vi "test_voltage.vi"() -> ()   [LabVIEW 2017]
panel:
  out "Det P (uW)":string
  out "Inc P (uW)":string
  out "Inc V (CORRECTED)":dbl
  out "Det V (CORRECTED)":dbl
  out "Det V / Inc V (CORRECTED)":dbl
  out "Incident Voltage (mV)":dbl
  out "Detected Voltage (mV)":dbl
  in  "Detected Offset":dbl
  in  "Incident Offset":dbl
  out "Det P / Inc P":dbl
  in  "number of samples":i32=100
  in  "rate":dbl=100.0
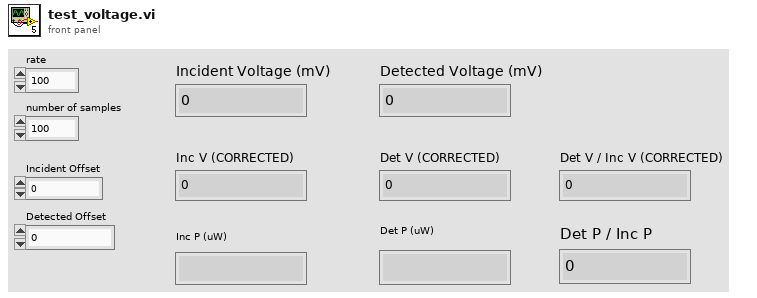
[diagram p1: front panel]
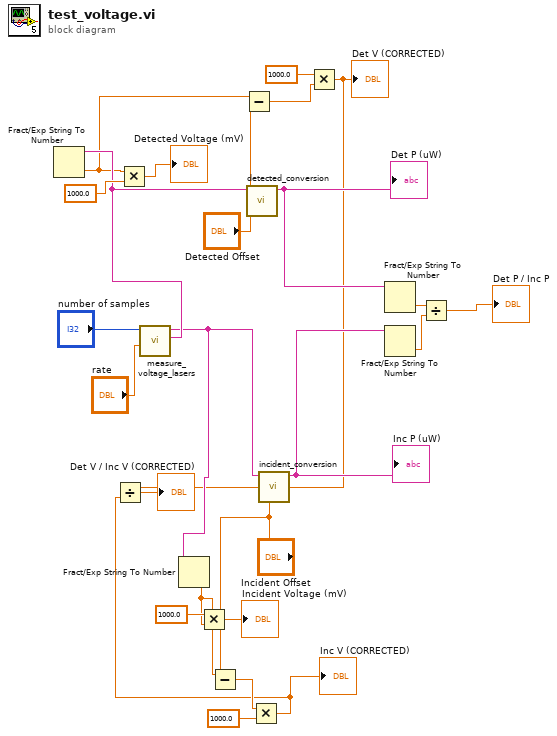
[diagram p0: block diagram]
diagram:
  n1 = call "measure_voltage_lasers.vi"("rate"="rate", "number of samples"="number of samples") -> ("Detected Voltage"=w16:string, "Incident Voltage"=w11:string)  [unwired: 6 in, 1 out]
  n2 = Fract/Exp String To Number(string=w16) -> (number=w10:dbl)  [unwired: 3 in, 1 out]
  n3 = Multiply(x=w10, y=1000.0) -> (x*y=→"Detected Voltage (mV)":dbl)
  n4 = Fract/Exp String To Number(string=w11) -> (number=w6:dbl)  [unwired: 3 in, 1 out]
  n5 = Multiply(x=1000.0, y=w6) -> (x*y=→"Incident Voltage (mV)":dbl)
  n6 = Subtract(x=w6, y="Incident Offset") -> (x-y=w4:dbl)
  n7 = Subtract(x=w10, y="Detected Offset") -> (x-y=w8:dbl)
  n8 = call "detected_conversion.vi"("Offset"="Detected Offset", "Voltage"=w16) -> ("Optical Power"=w18:string)  [unwired: 9 in]
  "Det P (uW)" <- w18
  n9 = Multiply(x=w4, y=1000.0) -> (x*y=w2:dbl)
  "Inc V (CORRECTED)" <- w2
  n10 = call "incident_conversion.vi"("Offset"="Incident Offset", "Voltage"=w11) -> ("Optical Power"=w19:string)  [unwired: 9 in]
  "Inc P (uW)" <- w19
  n11 = Multiply(x=1000.0, y=w8) -> (x*y=w1:dbl)
  "Det V (CORRECTED)" <- w1
  n12 = Divide(x=w1, y=w2) -> (x/y=→"Det V / Inc V (CORRECTED)":dbl)
  n13 = Fract/Exp String To Number(string=w18) -> (number=w22:dbl)  [unwired: 3 in, 1 out]
  n14 = Fract/Exp String To Number(string=w19) -> (number=w21:dbl)  [unwired: 3 in, 1 out]
  n15 = Divide(x=w22, y=w21) -> (x/y=→"Det P / Inc P":dbl)
